vi "write_data.vi"(0 "Data Folder":path, 1 "dP Data Prefix":string, 2 "dP Data Index":dbl, 3 "Data Labels":string[][](array[string])=[["Vap Mass Flow", "Liq Mass Flow", "DP", "Liq Tank P", "LiqTank T", "Sep P", "SepT", "Liq In P", "Liq In T", "Vap Tank P", "Vap Tank T", "Dev Section P", "Dev Section T", "Up TS P", "Up TS T", "Low TS P", "Low TS T", "Cond Top T", "Evap Top T", "Cond Bot T", "Evap Bot T", "Win 3-4 P", "Top Heat T", "Bot Heat T"]], 5 "dequeued data":dbl[][](array[numeric])) -> ()   [LabVIEW 2017]
uses:
  <vilib>/Utility/file.llb/Write Delimited Spreadsheet (DBL).vi
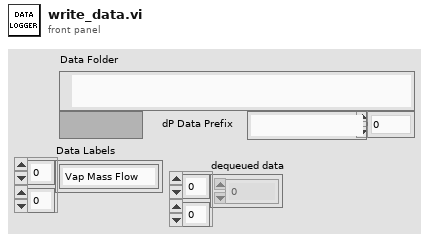
[diagram p1: front panel]
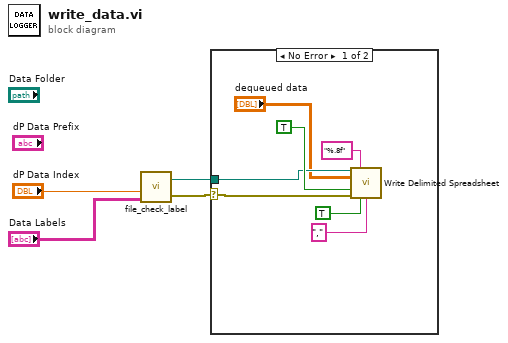
[diagram p0: block diagram]
diagram:
  n1 = call "file_check_label.vi"("Loop Data Labels"="Data Labels", "index"="dP Data Index") -> ("error out"=w1:errorcluster, "dup path"=w4:path)  [unwired: 4 in]
  n2 = case shown="No Error" w1 {
    selector: w1 -> [w5 _]
    tunnel: w4 -> [w8 _]
    frame No Error {
      n3 = call-poly <vilib>:"Write Delimited Spreadsheet.vi"("file path (dialog if empty)"=w8, "format (%.3f)"="%.8f", "2D data"="dequeued data", "append to file? (new file:F)"=TRUE ("append to file? (F)"), "error in (no error)"=w5, "transpose? (no:F)"=TRUE ("transpose? (F)"), "delimiter (\\t)"="," ("delimiter (\\t)")) -> ()  [unwired: 7 in, 2 out]
    }
    frame Error {
    }
  }
